vi "Format CSV.vi"(8 "error in (no error)":errorcluster, 9 "delimiter":string=",", 10 "CSV File Input":path, 11 "Original CSV Format":enum16{"Format A", "Format B"}(ring)) -> (0 "error out":errorcluster, 1 "Parcel Length":i32[](array[numeric]), 2 "All Terminal Data":T1(array[cluster]))   [LabVIEW 2017] (continued)
"30:40.9", "30:41.0", "30:41.0", "30:41.0", "30:41.1", "30:41.1", "30:41.1", "30:41.2", "30:41.2", "30:41.2", "30:41.3", "30:41.3", "30:41.3", "30:41.4", "30:41.4", "30:41.4", "30:41.5", "30:41.5", "30:41.5", "30:41.6", "30:41.6", "30:41.6", "30:41.7", "30:41.7", "30:41.7", "30:41.8", "30:41.8", "30:41.8", "30:41.9", "30:41.9", "30:41.9", "30:42.0", "30:42.0", "30:42.0", "30:42.1", "30:42.1", "30:42.1", "30:42.2", "30:42.2", "30:42.2", "30:42.3", "30:42.3", "30:42.3", "30:42.4", "30:42.4", "30:42.4", "30:42.5", "30:42.5", "30:42.5", "30:42.6", "30:42.6", "30:42.6", "30:42.7", "30:42.7", "30:42.7", "30:42.8", "30:42.8", "30:42.8", "30:42.9", "30:42.9", "30:42.9", "30:43.0", "30:43.0", "30:43.0", "30:43.1", "30:43.1", "30:43.1", "30:43.2", "30:43.2", "30:43.2", "30:43.3", "30:43.3", "30:43.3", "30:43.4", "30:43.4", "30:43.4", "30:43.5", "30:43.5", "30:43.5", "30:43.6", "30:43.6", "30:43.6", "30:43.7", "30:43.7", "30:43.7", "30:43.8", "30:43.8", "30:43.8", "30:43.9", "30:43.9", "30:43.9", "30:44.0", "30:44.0", "30:44.0", "30:44.1", "30:44.1", "30:44.1", "30:44.2", "30:44.2", "30:44.2", "30:44.3", "30:44.3", "30:44.3", "30:44.4", "30:44.4", "30:44.4", "30:44.5", "30:44.5", "30:44.5", "30:44.6", "30:44.6", "30:44.6", "30:44.7", "30:44.7", "30:44.7", "30:44.8", "30:44.8", "30:44.8", "30:44.9", "30:44.9", "30:44.9", "30:45.0", "30:45.0", "30:45.0", "30:45.1", "30:45.1", "30:45.1", "30:45.2", "30:45.2", "30:45.2", "30:45.3", "30:45.3", "30:45.3", "30:45.4", "30:45.4", "30:45.4", "30:45.5", "30:45.5", "30:45.5", "30:45.6", "30:45.6", "30:45.6", "30:45.7", "30:45.7", "30:45.7", "30:45.8", "30:45.8", "30:45.8", "30:45.9", "30:45.9", "30:45.9", "30:46.0", "30:46.0", "30:46.0", "30:46.1", "30:46.1", "30:46.1", "30:46.2", "30:46.2", "30:46.2", "30:46.3", "30:46.3", "30:46.3", "30:46.4", "30:46.4", "30:46.4", "30:46.5", "30:46.5", "30:46.5", "30:46.6", "30:46.6", "30:46.6", "30:46.7", "30:46.7", "30:46.7", "30:46.8", "30:46.8", "30:46.8", "30:46.9", "30:46.9", "30:46.9", "30:47.0", "30:47.0", "30:47.0", "30:47.1", "30:47.1", "30:47.1", "30:47.2", "30:47.2", "30:47.2", "30:47.3", "30:47.3", "30:47.3", "30:47.4", "30:47.4", "30:47.4", "30:47.5", "30:47.5", "30:47.5", "30:47.6", "30:47.6", "30:47.6", "30:47.7", "30:47.7", "30:47.7", "30:47.8", "30:47.8", "30:47.8", "30:47.9", "30:47.9", "30:47.9", "30:48.0", "30:48.0", "30:48.0", "30:48.1", "30:48.1", "30:48.1", "30:48.2", "30:48.2", "30:48.2", "30:48.3", "30:48.3", "30:48.3", "30:48.4", "30:48.4", "30:48.4", "30:48.5", "30:48.5", "30:48.5", "30:48.6", "30:48.6", "30:48.6", "30:48.7", "30:48.7", "30:48.7", "30:48.8", "30:48.8", "30:48.8", "30:48.9", "30:48.9", "30:48.9", "30:49.0", "30:49.0", "30:49.0", "30:49.1", "30:49.1", "30:49.1", "30:49.2", "30:49.2", "30:49.2", "30:49.3", "30:49.3", "30:49.3", "30:49.4", "30:49.4", "30:49.4", "30:49.5", "30:49.5", "30:49.5", "30:49.6", "30:49.6", "30:49.6", "30:49.7", "30:49.7", "30:49.7", "30:49.8", "30:49.8", "30:49.8", "30:49.9", "30:49.9", "30:49.9", "30:50.0", "30:50.0", "30:50.0", "30:50.1", "30:50.1", "30:50.1", "30:50.2", "30:50.2", "30:50.2", "30:50.3", "30:50.3", "30:50.3", "30:50.4", "30:50.4", "30:50.4", "30:50.5", "30:50.5", "30:50.5", "30:50.6", "30:50.6", "30:50.6", "30:50.7", "30:50.7", "30:50.7", "30:50.8", "30:50.8", "30:50.8", "30:50.9", "30:50.9", "30:50.9", "30:51.0", "30:51.0", "30:51.0", "30:51.1", "30:51.1", "30:51.1", "30:51.2", "30:51.2", "30:51.2", "30:51.3", "30:51.3", "30:51.3", "30:51.4", "30:51.4", "30:51.4", "30:51.5", "30:51.5", "30:51.5", "30:51.6", "30:51.6", "30:51.6", "30:51.7", "30:51.7", "30:51.7", "30:51.8", "30:51.8", "30:51.8", "30:51.9", "30:51.9", "30:51.9", "30:52.0", "30:52.0", "30:52.0", "30:52.1", "30:52.1", "30:52.1", "30:52.2", "30:52.2", "30:52.2", "30:52.3", "30:52.3", "30:52.3", "30:52.4", "30:52.4", "30:52.4", "30:52.5", "30:52.5", "30:52.5", "30:52.6", "30:52.6", "30:52.6", "30:52.7", "30:52.7", "30:52.7", "30:52.8", "30:52.8", "30:52.8", "30:52.9", "30:52.9", "30:52.9", "30:53.0", "30:53.0", "30:53.0", "30:53.1", "30:53.1", "30:53.1", "30:53.2", "30:53.2", "30:53.2", "30:53.3", "30:53.3", "30:53.3", "30:53.4", "30:53.4", "30:53.4", "30:53.5", "30:53.5", "30:53.5", "30:53.6", "30:53.6", "30:53.6", "30:53.7", "30:53.7", "30:53.7", "30:53.8", "30:53.8", "30:53.8", "30:53.9", "30:53.9", "30:53.9", "30:54.0", "30:54.0", "30:54.0", "30:54.1", "30:54.1", "30:54.1", "30:54.2", "30:54.2", "30:54.2", "30:54.3", "30:54.3", "30:54.3", "30:54.4", "30:54.4", "30:54.4", "30:54.5", "30:54.5", "30:54.5", "30:54.6", "30:54.6", "30:54.6", "30:54.7", "30:54.7", "30:54.7", "30:54.8", "30:54.8", "30:54.8", "30:54.9", "30:54.9", "30:54.9", "30:55.0", "30:55.0", "30:55.0", "30:55.1", "30:55.1", "30:55.1", "30:55.2", "30:55.2", "30:55.2", "30:55.3", "30:55.3", "30:55.3", "30:55.4", "30:55.4", "30:55.4", "30:55.5", "30:55.5", "30:55.5", "30:55.6", "30:55.6", "30:55.6", "30:55.7", "30:55.7", "30:55.7", "30:55.8", "30:55.8", "30:55.8", "30:55.9", "30:55.9", "30:55.9", "30:56.0", "30:56.0", "30:56.0", "30:56.1", "30:56.1", "30:56.1", "30:56.2", "30:56.2", "30:56.2", "30:56.3", "30:56.3", "30:56.3", "30:56.4", "30:56.4", "30:56.4", "30:56.5", "30:56.5", "30:56.5", "30:56.6", "30:56.6", "30:56.6", "30:56.7", "30:56.7", "30:56.7", "30:56.8", "30:56.8", "30:56.8", "30:56.9", "30:56.9", "30:56.9", "30:57.0", "30:57.0", "30:57.0", "30:57.1", "30:57.1", "30:57.1", "30:57.2", "30:57.2", "30:57.2", "30:57.3", "30:57.3", "30:57.3", "30:57.4", "30:57.4", "30:57.4", "30:57.5", "30:57.5", "30:57.5", "30:57.6", "30:57.6", "30:57.6", "30:57.7", "30:57.7", "30:57.7", "30:57.8", "30:57.8", "30:57.8", "30:57.9", "30:57.9", "30:57.9", "30:58.0", "30:58.0", "30:58.0", "30:58.1", "30:58.1", "30:58.1", "30:58.2", "30:58.2", "30:58.2", "30:58.3", "30:58.3", "30:58.3", "30:58.4", "30:58.4", "30:58.4", "30:58.5", "30:58.5", "30:58.5", "30:58.6", "30:58.6", "30:58.6", "30:58.7", "30:58.7", "30:58.7", "30:58.8", "30:58.8", "30:58.8", "30:58.9", "30:58.9", "30:58.9", "30:59.0", "30:59.0", "30:59.0", "30:59.1", "30:59.1", "30:59.1", "30:59.2", "30:59.2", "30:59.2", "30:59.3", "30:59.3", "30:59.3", "30:59.4", "30:59.4", "30:59.4", "30:59.5", "30:59.5", "30:59.5", "30:59.6", "30:59.6", "30:59.6", "30:59.7", "30:59.7", "30:59.7", "30:59.8", "30:59.8", "30:59.8", "30:59.9", "30:59.9", "30:59.9", "31:00.0", "31:00.0", "31:00.0", "31:00.1", "31:00.1", "31:00.1", "31:00.2", "31:00.2", "31:00.2", "31:00.3", "31:00.3", "31:00.3", "31:00.4", "31:00.4", "31:00.4", "31:00.5", "31:00.5", "31:00.5", "31:00.6", "31:00.6", "31:00.6", "31:00.7", "31:00.7", "31:00.7", "31:00.8", "31:00.8", "31:00.8", "31:00.9", "31:00.9", "31:00.9", "31:01.0", "31:01.0", "31:01.0", "31:01.1", "31:01.1", "31:01.1", "31:01.2", "31:01.2", "31:01.2", "31:01.3", "31:01.3", "31:01.3", "31:01.4", "31:01.4", "31:01.4", "31:01.5", "31:01.5", "31:01.5", "31:01.6", "31:01.6", "31:01.6", "31:01.7", "31:01.7", "31:01.7", "31:01.8", "31:01.8", "31:01.8", "31:01.9", "31:01.9", "31:01.9", "31:02.0", "31:02.0", "31:02.0", "31:02.1", "31:02.1", "31:02.1", "31:02.2", "31:02.2", "31:02.2", "31:02.3", "31:02.3", "31:02.3", "31:02.4", "31:02.4", "31:02.4", "31:02.5", "31:02.5", "31:02.5", "31:02.6", "31:02.6", "31:02.6", "31:02.7", "31:02.7", "31:02.7", "31:02.8", "31:02.8", "31:02.8", "31:02.9", "31:02.9", "31:02.9", "31:03.0", "31:03.0", "31:03.0", "31:03.1", "31:03.1", "31:03.1", "31:03.2", "31:03.2", "31:03.2", "31:03.3", "31:03.3", "31:03.3", "31:03.4", "31:03.4", "31:03.4", "31:03.5", "31:03.5", "31:03.5", "31:03.6", "31:03.6", "31:03.6", "31:03.7", "31:03.7", "31:03.7", "31:03.8", "31:03.8", "31:03.8", "31:03.9", "31:03.9", "31:03.9", "31:04.0", "31:04.0", "31:04.0", "31:04.1", "31:04.1", "31:04.1", "31:04.2", "31:04.2", "31:04.2", "31:04.3", "31:04.3", "31:04.3", "31:04.4", "31:04.4", "31:04.4", "31:04.5", "31:04.5", "31:04.5", "31:04.6", "31:04.6", "31:04.6", "31:04.7", "31:04.7", "31:04.7", "31:04.8", "31:04.8", "31:04.8", "31:04.9", "31:04.9", "31:04.9", "31:05.0", "31:05.0", "31:05.0", "31:05.1", "31:05.1", "31:05.1", "31:05.2", "31:05.2", "31:05.2", "31:05.3", "31:05.3", "31:05.3", "31:05.4", "31:05.4", "31:05.4", "31:05.5", "31:05.5", "31:05.5", "31:05.6", "31:05.6", "31:05.6", "31:05.7", "31:05.7", "31:05.7", "31:05.8", "31:05.8", "31:05.8", "31:05.9", "31:05.9", "31:05.9", "31:06.0", "31:06.0", "31:06.0", "31:06.1", "31:06.1", "31:06.1", "31:06.2", "31:06.2", "31:06.2", "31:06.3", "31:06.3", "31:06.3", "31:06.4", "31:06.4", "31:06.4", "31:06.5", "31:06.5", "31:06.5", "31:06.6", "31:06.6", "31:06.6", "31:06.7", "31:06.7", "31:06.7", "31:06.8", "31:06.8", "31:06.8", "31:06.9", "31:06.9", "31:06.9", "31:07.0", "31:07.0", "31:07.0", "31:07.1", "31:07.1", "31:07.1", "31:07.2", "31:07.2", "31:07.2", "31:07.3", "31:07.3", "31:07.3", "31:07.4", "31:07.4", "31:07.4", "31:07.5", "31:07.5", "31:07.5", "31:07.6", "31:07.6", "31:07.6", "31:07.7", "31:07.7", "31:07.7", "31:07.8", "31:07.8", "31:07.8", "31:07.9", "31:07.9", "31:07.9", "31:08.0", "31:08.0", "31:08.0", "31:08.1", "31:08.1", "31:08.1", "31:08.2", "31:08.2", "31:08.2", "31:08.3", "31:08.3", "31:08.3", "31:08.4", "31:08.4", "31:08.4", "31:08.5", "31:08.5", "31:08.5", "31:08.6", "31:08.6", "31:08.6", "31:08.7", "31:08.7", "31:08.7", "31:08.8", "31:08.8", "31:08.8", "31:08.9", "31:08.9", "31:08.9", "31:09.0", "31:09.0", "31:09.0", "31:09.1", "31:09.1", "31:09.1", "31:09.2", "31:09.2", "31:09.2", "31:09.3", "31:09.3", "31:09.3", "31:09.4", "31:09.4", "31:09.4", "31:09.5", "31:09.5", "31:09.5", "31:09.6", "31:09.6", "31:09.6", "31:09.7", "31:09.7", "31:09.7", "31:09.8", "31:09.8", "31:09.8", "31:09.9", "31:09.9", "31:09.9", "31:10.0", "31:10.0", "31:10.0", "31:10.1", "31:10.1", "31:10.1", "31:10.2", "31:10.2", "31:10.2", "31:10.3", "31:10.3", "31:10.3", "31:10.4", "31:10.4", "31:10.4", "31:10.5", "31:10.5", "31:10.5", "31:10.6", "31:10.6", "31:10.6", "31:10.7", "31:10.7", "31:10.7", "31:10.8", "31:10.8", "31:10.8", "31:10.9", "31:10.9", "31:10.9", "31:11.0", "31:11.0", "31:11.0", "31:11.1", "31:11.1", "31:11.1", "31:11.2", "31:11.2", "31:11.2", "31:11.3", "31:11.3", "31:11.3", "31:11.4", "31:11.4", "31:11.4", "31:11.5", "31:11.5", "31:11.5", "31:11.6", "31:11.6", "31:11.6", "31:11.7", "31:11.7", "31:11.7", "31:11.8", "31:11.8", "31:11.8", "31:11.9", "31:11.9", "31:11.9", "31:12.0", "31:12.0", "31:12.0", "31:12.1", "31:12.1", "31:12.1", "31:12.2", "31:12.2", "31:12.2", "31:12.3", "31:12.3", "31:12.3", "31:12.4", "31:12.4", "31:12.4", "31:12.5", "31:12.5", "31:12.5", "31:12.6", "31:12.6", "31:12.6", "31:12.7", "31:12.7", "31:12.7", "31:12.8", "31:12.8", "31:12.8", "31:12.9", "31:12.9", "31:12.9", "31:13.0", "31:13.0", "31:13.0", "31:13.1", "31:13.1", "31:13.1", "31:13.2", "31:13.2", "31:13.2", "31:13.3", "31:13.3", "31:13.3", "31:13.4", "31:13.4", "31:13.4", "31:13.5", "31:13.5", "31:13.5", "31:13.6", "31:13.6", "31:13.6", "31:13.7", "31:13.7", "31:13.7", "31:13.8", "31:13.8", "31:13.8", "31:13.9", "31:13.9", "31:13.9", "31:14.0", "31:14.0", "31:14.0", "31:14.1", "31:14.1", "31:14.1", "31:14.2", "31:14.2", "31:14.2", "31:14.3", "31:14.3", "31:14.3", "31:14.4", "31:14.4", "31:14.4", "31:14.5", "31:14.5", "31:14.5", "31:14.6", "31:14.6", "31:14.6", "31:14.7", "31:14.7", "31:14.7", "31:14.8", "31:14.8", "31:14.8", "31:14.9", "31:14.9", "31:14.9", "31:15.0", "31:15.0", "31:15.0", "31:15.1", "31:15.1", "31:15.1", "31:15.2", "31:15.2", "31:15.2", "31:15.3", "31:15.3", "31:15.3", "31:15.4", "31:15.4", "31:15.4", "31:15.5", "31:15.5", "31:15.5", "31:15.6", "31:15.6", "31:15.6", "31:15.7", "31:15.7", "31:15.7", "31:15.8", "31:15.8", "31:15.8", "31:15.9", "31:15.9", "31:15.9", "31:16.0", "31:16.0", "31:16.0", "31:16.1", "31:16.1", "31:16.1", "31:16.2", "31:16.2", "31:16.2", "31:16.3", "31:16.3", "31:16.3", "31:16.4", "31:16.4", "31:16.4", "31:16.5", "31:16.5", "31:16.5", "31:16.6", "31:16.6", "31:16.6", "31:16.7", "31:16.7", "31:16.7", "31:16.8", "31:16.8", "31:16.8", "31:16.9", "31:16.9", "31:16.9", "31:17.0", "31:17.0", "31:17.0", "31:17.1", "31:17.1", "31:17.1", "31:17.2", "31:17.2", "31:17.2", "31:17.3", "31:17.3", "31:17.3", "31:17.4", "31:17.4", "31:17.4", "31:17.5", "31:17.5", "31:17.5", "31:17.6", "31:17.6", "31:17.6", "31:17.7", "31:17.7", "31:17.7", "31:17.8", "31:17.8", "31:17.8", "31:17.9", "31:17.9", "31:17.9", "31:18.0", "31:18.0", "31:18.0", "31:18.1", "31:18.1", "31:18.1", "31:18.2", "31:18.2", "31:18.2", "31:18.3", "31:18.3", "31:18.3", "31:18.4", "31:18.4", "31:18.4", "31:18.5", "31:18.5", "31:18.5", "31:18.6", "31:18.6", "31:18.6", "31:18.7", "31:18.7", "31:18.7", "31:18.8", "31:18.8", "31:18.8", "31:18.9", "31:18.9", "31:18.9", "31:19.0", "31:19.0", "31:19.0", "31:19.1", "31:19.1", "31:19.1", "31:19.2", "31:19.2", "31:19.2", "31:19.3", "31:19.3", "31:19.3", "31:19.4", "31:19.4", "31:19.4", "31:19.5", "31:19.5", "31:19.5", "31:19.6", "31:19.6", "31:19.6", "31:19.7", "31:19.7", "31:19.7", "31:19.8", "31:19.8", "31:19.8", "31:19.9", "31:19.9", "31:19.9", "31:20.0", "31:20.0", "31:20.0", "31:20.1", "31:20.1", "31:20.1", "31:20.2", "31:20.2", "31:20.2", "31:20.3", "31:20.3", "31:20.3", "31:20.4", "31:20.4", "31:20.4", "31:20.5", "31:20.5", "31:20.5", "31:20.6", "31:20.6", "31:20.6", "31:20.7", "31:20.7", "31:20.7", "31:20.8", "31:20.8", "31:20.8", "31:20.9", "31:20.9", "31:20.9", "31:21.0", "31:21.0", "31:21.0", "31:21.1", "31:21.1", "31:21.1", "31:21.2", "31:21.2", "31:21.2", "31:21.3", "31:21.3", "31:21.3", "31:21.4", "31:21.4", "31:21.4", "31:21.5", "31:21.5", "31:21.5", "31:21.6", "31:21.6", "31:21.6", "31:21.7", "31:21.7", "31:21.7", "31:21.8", "31:21.8", "31:21.8", "31:21.9", "31:21.9", "31:21.9", "31:22.0", "31:22.0", "31:22.0", "31:22.1", "31:22.1", "31:22.1", "31:22.2", "31:22.2", "31:22.2", "31:22.3", "31:22.3", "31:22.3", "31:22.4", "31:22.4", "31:22.4", "31:22.5", "31:22.5", "31:22.5", "31:22.6", "31:22.6", "31:22.6", "31:22.7", "31:22.7", "31:22.7", "31:22.8", "31:22.8", "31:22.8", "31:22.9", "31:22.9", "31:22.9", "31:23.0", "31:23.0", "31:23.0", "31:23.1", "31:23.1", "31:23.1", "31:23.2", "31:23.2", "31:23.2", "31:23.3", "31:23.3", "31:23.3", "31:23.4", "31:23.4", "31:23.4", "31:23.5", "31:23.5", "31:23.5", "31:23.6", "31:23.6", "31:23.6", "31:23.7", "31:23.7", "31:23.7", "31:23.8", "31:23.8", "31:23.8", "31:23.9", "31:23.9", "31:23.9", "31:24.0", "31:24.0", "31:24.0", "31:24.1", "31:24.1", "31:24.1", "31:24.2", "31:24.2", "31:24.2", "31:24.3", "31:24.3", "31:24.3", "31:24.4", "31:24.4", "31:24.4", "31:24.5", "31:24.5", "31:24.5", "31:24.6", "31:24.6", "31:24.6", "31:24.7", "31:24.7", "31:24.7", "31:24.8", "31:24.8", "31:24.8", "31:24.9", "31:24.9", "31:24.9", "31:25.0", "31:25.0", "31:25.0", "31:25.1", "31:25.1", "31:25.1", "31:25.2", "31:25.2", "31:25.2", "31:25.3", "31:25.3", "31:25.3", "31:25.4", "31:25.4", "31:25.4", "31:25.5", "31:25.5", "31:25.5", "31:25.6", "31:25.6", "31:25.6", "31:25.7", "31:25.7", "31:25.7", "31:25.8", "31:25.8", "31:25.8", "31:25.9", "31:25.9", "31:25.9", "31:26.0", "31:26.0", "31:26.0", "31:26.1", "31:26.1", "31:26.1", "31:26.2", "31:26.2", "31:26.2", "31:26.3", "31:26.3", "31:26.3", "31:26.4", "31:26.4", "31:26.4", "31:26.5", "31:26.5", "31:26.5", "31:26.6", "31:26.6", "31:26.6", "31:26.7", "31:26.7", "31:26.7", "31:26.8", "31:26.8", "31:26.8", "31:26.9", "31:26.9", "31:26.9", "31:27.0", "31:27.0", "31:27.0", "31:27.1", "31:27.1", "31:27.1", "31:27.2", "31:27.2", "31:27.2", "31:27.3", "31:27.3", "31:27.3", "31:27.4", "31:27.4", "31:27.4", "31:27.5", "31:27.5", "31:27.5", "31:27.6", "31:27.6", "31:27.6", "31:27.7", "31:27.7", "31:27.7", "31:27.8", "31:27.8", "31:27.8", "31:27.9", "31:27.9", "31:27.9", "31:28.0", "31:28.0", "31:28.0", "31:28.1", "31:28.1", "31:28.1", "31:28.2", "31:28.2", "31:28.2", "31:28.3", "31:28.3", "31:28.3", "31:28.4", "31:28.4", "31:28.4", "31:28.5", "31:28.5", "31:28.5", "31:28.6", "31:28.6", "31:28.6", "31:28.7", "31:28.7", "31:28.7", "31:28.8", "31:28.8", "31:28.8", "31:28.9", "31:28.9", "31:28.9", "31:29.0", "31:29.0", "31:29.0", "31:29.1", "31:29.1", "31:29.1", "31:29.2", "31:29.2", "31:29.2", "31:29.3", "31:29.3", "31:29.3", "31:29.4", "31:29.4", "31:29.4", "31:29.5", "31:29.5", "31:29.5", "31:29.6", "31:29.6", "31:29.6", "31:29.7", "31:29.7", "31:29.7", "31:29.8", "31:29.8", "31:29.8", "31:29.9", "31:29.9", "31:29.9", "31:30.0", "31:30.0", "31:30.0", "31:30.1", "31:30.1", "31:30.1", "31:30.2", "31:30.2", "31:30.2", "31:30.3", "31:30.3", "31:30.3", "31:30.4", "31:30.4", "31:30.4", "31:30.5", "31:30.5", "31:30.5", "31:30.6", "31:30.6", "31:30.6", "31:30.7", "31:30.7", "31:30.7", "31:30.8", "31:30.8", "31:30.8", "31:30.9", "31:30.9", "31:30.9", "31:31.0", "31:31.0", "31:31.0", "31:31.1", "31:31.1", "31:31.1", "31:31.2", "31:31.2", "31:31.2", "31:31.3", "31:31.3", "31:31.3", "31:31.4", "31:31.4", "31:31.4", "31:31.5", "31:31.5", "31:31.5", "31:31.6", "31:31.6", "31:31.6", "31:31.7", "31:31.7", "31:31.7", "31:31.8", "31:31.8", "31:31.8", "31:31.9", "31:31.9", "31:31.9", "31:32.0", "31:32.0", "31:32.0", "31:32.1", "31:32.1", "31:32.1", "31:32.2", "31:32.2", "31:32.2", "31:32.3", "31:32.3", "31:32.3", "31:32.4", "31:32.4", "31:32.4", "31:32.5", "31:32.5", "31:32.5", "31:32.6", "31:32.6", "31:32.6", "31:32.7", "31:32.7", "31:32.7", "31:32.8", "31:32.8", "31:32.8", "31:32.9", "31:32.9", "31:32.9", "31:33.0", "31:33.0", "31:33.0", "31:33.1", "31:33.1", "31:33.1", "31:33.2", "31:33.2", "31:33.2", "31:33.3", "31:33.3", "31:33.3", "31:33.4", "31:33.4", "31:33.4", "31:33.5", "31:33.5", "31:33.5", "31:33.6", "31:33.6", "31:33.6", "31:33.7", "31:33.7", "31:33.7", "31:33.8", "31:33.8", "31:33.8", "31:33.9", "31:33.9", "31:33.9", "31:34.0", "31:34.0", "31:34.0", "31:34.1", "31:34.1", "31:34.1", "31:34.2", "31:34.2", "31:34.2", "31:34.3", "31:34.3", "31:34.3", "31:34.4", "31:34.4", "31:34.4", "31:34.5", "31:34.5", "31:34.5", "31:34.6", "31:34.6", "31:34.6", "31:34.7", "31:34.7", "31:34.7", "31:34.8", "31:34.8", "31:34.8", "31:34.9", "31:34.9", "31:34.9", "31:35.0", "31:35.0", "31:35.0", "31:35.1", "31:35.1", "31:35.1", "31:35.2", "31:35.2", "31:35.2", "31:35.3", "31:35.3", "31:35.3", "31:35.4", "31:35.4", "31:35.4", "31:35.5", "31:35.5", "31:35.5", "31:35.6", "31:35.6", "31:35.6", "31:35.7", "31:35.7", "31:35.7", "31:35.8", "31:35.8", "31:35.8", "31:35.9", "31:35.9", "31:35.9", "31:36.0", "31:36.0", "31:36.0", "31:36.1", "31:36.1", "31:36.1", "31:36.2", "31:36.2", "31:36.2", "31:36.3", "31:36.3", "31:36.3", "31:36.4", "31:36.4", "31:36.4", "31:36.5", "31:36.5", "31:36.5", "31:36.6", "31:36.6", "31:36.6", "31:36.7", "31:36.7", "31:36.7", "31:36.8", "31:36.8", "31:36.8", "31:36.9", "31:36.9", "31:36.9", "31:37.0", "31:37.0", "31:37.0", "31:37.1", "31:37.1", "31:37.1", "31:37.2", "31:37.2", "31:37.2", "31:37.3", "31:37.3", "31:37.3", "31:37.4", "31:37.4", "31:37.4", "31:37.5", "31:37.5", "31:37.5", "31:37.6", "31:37.6", "31:37.6", "31:37.7", "31:37.7", "31:37.7", "31:37.8", "31:37.8", "31:37.8", "31:37.9", "31:37.9", "31:37.9", "31:38.0", "31:38.0", "31:38.0", "31:38.1", "31:38.1", "31:38.1", "31:38.2", "31:38.2", "31:38.2", "31:38.3", "31:38.3", "31:38.3", "31:38.4", "31:38.4", "31:38.4", "31:38.5", "31:38.5", "31:38.5", "31:38.6", "31:38.6", "31:38.6", "31:38.7", "31:38.7", "31:38.7", "31:38.8", "31:38.8", "31:38.8", "31:38.9", "31:38.9", "31:38.9", "31:39.0", "31:39.0", "31:39.0", "31:39.1", "31:39.1", "31:39.1", "31:39.2", "31:39.2", "31:39.2", "31:39.3", "31:39.3", "31:39.3", "31:39.4", "31:39.4", "31:39.4", "31:39.5", "31:39.5", "31:39.5", "31:39.6", "31:39.6", "31:39.6", "31:39.7", "31:39.7", "31:39.7", "31:39.8", "31:39.8", "31:39.8", "31:39.9", "31:39.9", "31:39.9", "31:40.0", "31:40.0", "31:40.0", "31:40.1", "31:40.1", "31:40.1", "31:40.2", "31:40.2", "31:40.2", "31:40.3", "31:40.3", "31:40.3", "31:40.4", "31:40.4", "31:40.4", "31:40.5", "31:40.5", "31:40.5", "31:40.6", "31:40.6", "31:40.6", "31:40.7", "31:40.7", "31:40.7", "31:40.8", "31:40.8", "31:40.8", "31:40.9", "31:40.9", "31:40.9", "31:41.0", "31:41.0", "31:41.0", "31:41.1", "31:41.1", "31:41.1", "31:41.2", "31:41.2", "31:41.2", "31:41.3", "31:41.3", "31:41.3", "31:41.4", "31:41.4", "31:41.4", "31:41.5", "31:41.5", "31:41.5", "31:41.6", "31:41.6", "31:41.6", "31:41.7", "31:41.7", "31:41.7", "31:41.8", "31:41.8", "31:41.8", "31:41.9", "31:41.9", "31:41.9", "31:42.0", "31:42.0", "31:42.0", "31:42.1", "31:42.1", "31:42.1", "31:42.2", "31:42.2", "31:42.2", "31:42.3", "31:42.3", "31:42.3", "31:42.4", "31:42.4", "31:42.4", "31:42.5", "31:42.5", "31:42.5", "31:42.6", "31:42.6", "31:42.6", "31:42.7", "31:42.7", "31:42.7", "31:42.8", "31:42.8", "31:42.8", "31:42.9", "31:42.9", "31:42.9", "31:43.0", "31:43.0", "31:43.0", "31:43.1", "31:43.1", "31:43.1", "31:43.2", "31:43.2", "31:43.2", "31:43.3", "31:43.3", "31:43.3", "31:43.4", "31:43.4", "31:43.4", "31:43.5", "31:43.5", "31:43.5", "31:43.6", "31:43.6", "31:43.6", "31:43.7", "31:43.7", "31:43.7", "31:43.8", "31:43.8", "31:43.8", "31:43.9", "31:43.9", "31:43.9", "31:44.0", "31:44.0", "31:44.0", "31:44.1", "31:44.1", "31:44.1", "31:44.2", "31:44.2", "31:44.2", "31:44.3", "31:44.3", "31:44.3", "31:44.4", "31:44.4", "31:44.4", "31:44.5", "31:44.5", "31:44.5", "31:44.6", "31:44.6", "31:44.6", "31:44.7", "31:44.7", "31:44.7", "31:44.8", "31:44.8", "31:44.8", "31:44.9", "31:44.9", "31:44.9", "31:45.0", "31:45.0", "31:45.0", "31:45.1", "31:45.1", "31:45.1", "31:45.2", "31:45.2", "31:45.2", "31:45.3", "31:45.3", "31:45.3", "31:45.4", "31:45.4", "31:45.4", "31:45.5", "31:45.5", "31:45.5", "31:45.6", "31:45.6", "31:45.6", "31:45.7", "31:45.7", "31:45.7", "31:45.8", "31:45.8", "31:45.8", "31:45.9", "31:45.9", "31:45.9", "31:46.0", "31:46.0", "31:46.0", "31:46.1", "31:46.1", "31:46.1", "31:46.2", "31:46.2", "31:46.2", "31:46.3", "31:46.3", "31:46.3", "31:46.4", "31:46.4", "31:46.4", "31:46.5", "31:46.5", "31:46.5", "31:46.6", "31:46.6", "31:46.6", "31:46.7", "31:46.7", "31:46.7", "31:46.8", "31:46.8", "31:46.8", "31:46.9", "31:46.9", "31:46.9", "31:47.0", "31:47.0", "31:47.0", "31:47.1", "31:47.1", "31:47.1", "31:47.2", "31:47.2", "31:47.2", "31:47.3", "31:47.3", "31:47.3", "31:47.4", "31:47.4", "31:47.4", "31:47.5", "31:47.5", "31:47.5", "31:47.6", "31:47.6", "31:47.6", "31:47.7", "31:47.7", "31:47.7", "31:47.8", "31:47.8", "31:47.8", "31:47.9", "31:47.9", "31:47.9", "31:48.0", "31:48.0", "31:48.0", "31:48.1", "31:48.1", "31:48.1", "31:48.2", "31:48.2", "31:48.2", "31:48.3", "31:48.3", "31:48.3", "31:48.4", "31:48.4", "31:48.4", "31:48.5", "31:48.5", "31:48.5", "31:48.6", "31:48.6", "31:48.6", "31:48.7", "31:48.7", "31:48.7", "31:48.8", "31:48.8", "31:48.8", "31:48.9", "31:48.9", "31:48.9", "31:49.0", "31:49.0", "31:49.0", "31:49.1", "31:49.1", "31:49.1", "31:49.2", "31:49.2", "31:49.2", "31:49.3", "31:49.3", "31:49.3", "31:49.4", "31:49.4", "31:49.4", "31:49.5", "31:49.5", "31:49.5", "31:49.6", "31:49.6", "31:49.6", "31:49.7", "31:49.7", "31:49.7", "31:49.8", "31:49.8", "31:49.8", "31:49.9", "31:49.9", "31:49.9", "31:50.0", "31:50.0", "31:50.0", "31:50.1", "31:50.1", "31:50.1", "31:50.2", "31:50.2", "31:50.2", "31:50.3", "31:50.3", "31:50.3", "31:50.4", "31:50.4", "31:50.4", "31:50.5", "31:50.5", "31:50.5", "31:50.6", "31:50.6", "31:50.6", "31:50.7", "31:50.7", "31:50.7", "31:50.8", "31:50.8", "31:50.8", "31:50.9", "31:50.9", "31:50.9", "31:51.0", "31:51.0", "31:51.0", "31:51.1", "31:51.1", "31:51.1", "31:51.2", "31:51.2", "31:51.2", "31:51.3", "31:51.3", "31:51.3", "31:51.4", "31:51.4", "31:51.4", "31:51.5", "31:51.5", "31:51.5", "31:51.6", "31:51.6", "31:51.6", "31:51.7", "31:51.7", "31:51.7", "31:51.8", "31:51.8", "31:51.8", "31:51.9", "31:51.9", "31:51.9", "31:52.0", "31:52.0", "31:52.0", "31:52.1", "31:52.1", "31:52.1", "31:52.2", "31:52.2", "31:52.2", "31:52.3", "31:52.3", "31:52.3", "31:52.4", "31:52.4", "31:52.4", "31:52.5", "31:52.5", "31:52.5", "31:52.6", "31:52.6", "31:52.6", "31:52.7", "31:52.7", "31:52.7", "31:52.8", "31:52.8", "31:52.8", "31:52.9", "31:52.9", "31:52.9", "31:53.0", "31:53.0", "31:53.0", "31:53.1", "31:53.1", "31:53.1", "31:53.2", "31:53.2", "31:53.2", "31:53.3", "31:53.3", "31:53.3", "31:53.4", "31:53.4", "31:53.4", "31:53.5", "31:53.5", "31:53.5", "31:53.6", "31:53.6", "31:53.6", "31:53.7", "31:53.7", "31:53.7", "31:53.8", "31:53.8", "31:53.8", "31:53.9", "31:53.9", "31:53.9", "31:54.0", "31:54.0", "31:54.0", "31:54.1", "31:54.1", "31:54.1", "31:54.2", "31:54.2", "31:54.2", "31:54.3", "31:54.3", "31:54.3", "31:54.4", "31:54.4", "31:54.4", "31:54.5", "31:54.5", "31:54.5", "31:54.6", "31:54.6", "31:54.6", "31:54.7", "31:54.7", "31:54.7", "31:54.8", "31:54.8", "31:54.8", "31:54.9", "31:54.9", "31:54.9", "31:55.0", "31:55.0", "31:55.0", "31:55.1", "31:55.1", "31:55.1", "31:55.2", "31:55.2", "31:55.2", "31:55.3", "31:55.3", "31:55.3", "31:55.4", "31:55.4", "31:55.4", "31:55.5", "31:55.5", "31:55.5", "31:55.6", "31:55.6", "31:55.6", "31:55.7", "31:55.7", "31:55.7", "31:55.8", "31:55.8", "31:55.8", "31:55.9", "31:55.9", "31:55.9", "31:56.0", "31:56.0", "31:56.0", "31:56.1", "31:56.1", "31:56.1", "31:56.2", "31:56.2", "31:56.2", "31:56.3", "31:56.3", "31:56.3", "31:56.4", "31:56.4", "31:56.4", "31:56.5", "31:56.5", "31:56.5", "31:56.6", "31:56.6", "31:56.6", "31:56.7", "31:56.7", "31:56.7", "31:56.8", "31:56.8", "31:56.8", "31:56.9", "31:56.9", "31:56.9", "31:57.0", "31:57.0", "31:57.0", "31:57.1", "31:57.1", "31:57.1", "31:57.2", "31:57.2", "31:57.2", "31:57.3", "31:57.3", "31:57.3", "31:57.4", "31:57.4", "31:57.4", "31:57.5", "31:57.5", "31:57.5", "31:57.6", "31:57.6", "31:57.6", "31:57.7", "31:57.7", "31:57.7", "31:57.8", "31:57.8", "31:57.8", "31:57.9", "31:57.9", "31:57.9", "31:58.0", "31:58.0", "31:58.0", "31:58.1", "31:58.1", "31:58.1", "31:58.2", "31:58.2", "31:58.2", "31:58.3", "31:58.3", "31:58.3", "31:58.4", "31:58.4", "31:58.4", "31:58.5", "31:58.5", "31:58.5", "31:58.6", "31:58.6", "31:58.6", "31:58.7", "31:58.7", "31:58.7", "31:58.8", "31:58.8", "31:58.8", "31:58.9", "31:58.9", "31:58.9", "31:59.0", "31:59.0", "31:59.0", "31:59.1", "31:59.1", "31:59.1", "31:59.2", "31:59.2", "31:59.2", "31:59.3", "31:59.3", "31:59.3", "31:59.4", "31:59.4", "31:59.4", "31:59.5", "31:59.5", "31:59.5", "31:59.6", "31:59.6", "31:59.6", "31:59.7", "31:59.7", "31:59.7", "31:59.8", "31:59.8", "31:59.8", "31:59.9", "31:59.9", "31:59.9", "32:00.0", "32:00.0", "32:00.0", "32:00.1", "32:00.1", "32:00.1", "32:00.2", "32:00.2", "32:00.2", "32:00.3", "32:00.3", "32:00.3", "32:00.4", "32:00.4", "32:00.4", "32:00.5", "32:00.5", "32:00.5", "32:00.6", "32:00.6", "32:00.6", "32:00.7", "32:00.7", "32:00.7", "32:00.8", "32:00.8", "32:00.8", "32:00.9", "32:00.9", "32:00.9", "32:01.0", "32:01.0", "32:01.0", "32:01.1", "32:01.1", "32:01.1", "32:01.2", "32:01.2", "32:01.2", "32:01.3", "32:01.3", "32:01.3", "32:01.4", "32:01.4", "32:01.4", "32:01.5", "32:01.5", "32:01.5", "32:01.6", "32:01.6", "32:01.6", "32:01.7", "32:01.7", "32:01.7", "32:01.8", "32:01.8", "32:01.8", "32:01.9", "32:01.9", "32:01.9", "32:02.0", "32:02.0", "32:02.0", "32:02.1", "32:02.1", "32:02.1", "32:02.2", "32:02.2", "32:02.2", "32:02.3", "32:02.3", "32:02.3", "32:02.4", "32:02.4", "32:02.4", "32:02.5", "32:02.5", "32:02.5", "32:02.6", "32:02.6", "32:02.6", "32:02.7", "32:02.7", "32:02.7", "32:02.8", "32:02.8", "32:02.8", "32:02.9", "32:02.9", "32:02.9", "32:03.0", "32:03.0", "32:03.0", "32:03.1", "32:03.1", "32:03.1", "32:03.2", "32:03.2", "32:03.2", "32:03.3", "32:03.3", "32:03.3", "32:03.4", "32:03.4", "32:03.4", "32:03.5", "32:03.5", "32:03.5", "32:03.6", "32:03.6", "32:03.6", "32:03.7", "32:03.7", "32:03.7", "32:03.8", "32:03.8", "32:03.8", "32:03.9", "32:03.9", "32:03.9", "32:04.0", "32:04.0", "32:04.0", "32:04.1", "32:04.1", "32:04.1", "32:04.2", "32:04.2", "32:04.2", "32:04.3", "32:04.3", "32:04.3", "32:04.4", "32:04.4", "32:04.4", "32:04.5", "32:04.5", "32:04.5", "32:04.6", "32:04.6", "32:04.6", "32:04.7", "32:04.7", "32:04.7", "32:04.8", "32:04.8", "32:04.8", "32:04.9", "32:04.9", "32:04.9", "32:05.0", "32:05.0", "32:05.0", "32:05.1", "32:05.1", "32:05.1", "32:05.2", "32:05.2", "32:05.2", "32:05.3", "32:05.3", "32:05.3", "32:05.4", "32:05.4", "32:05.4", "32:05.5", "32:05.5", "32:05.5", "32:05.6", "32:05.6", "32:05.6", "32:05.7", "32:05.7", "32:05.7", "32:05.8", "32:05.8", "32:05.8", "32:05.9", "32:05.9", "32:05.9", "32:06.0", "32:06.0", "32:06.0", "32:06.1", "32:06.1", "32:06.1", "32:06.2", "32:06.2", "32:06.2", "32:06.3", "32:06.3", "32:06.3", "32:06.4", "32:06.4", "32:06.4", "32:06.5", "32:06.5", "32:06.5", "32:06.6", "32:06.6", "32:06.6", "32:06.7", "32:06.7", "32:06.7", "32:06.8", "32:06.8", "32:06.8", "32:06.9", "32:06.9", "32:06.9", "32:07.0", "32:07.0", "32:07.0", "32:07.1", "32:07.1", "32:07.1", "32:07.2", "32:07.2", "32:07.2", "32:07.3", "32:07.3", "32:07.3", "32:07.4", "32:07.4", "32:07.4", "32:07.5", "32:07.5", "32:07.5", "32:07.6", "32:07.6", "32:07.6", "32:07.7", "32:07.7", "32:07.7", "32:07.8", "32:07.8", "32:07.8", "32:07.9", "32:07.9", "32:07.9", "32:08.0", "32:08.0", "32:08.0", "32:08.1", "32:08.1", "32:08.1", "32:08.2", "32:08.2", "32:08.2", "32:08.3", "32:08.3", "32:08.3", "32:08.4", "32:08.4", "32:08.4", "32:08.5", "32:08.5", "32:08.5", "32:08.6", "32:08.6", "32:08.6", "32:08.7", "32:08.7", "32:08.7", "32:08.8", "32:08.8", "32:08.8", "32:08.9", "32:08.9", "32:08.9", "32:09.0", "32:09.0", "32:09.0", "32:09.1", "32:09.1", "32:09.1", "32:09.2", "32:09.2", "32:09.2", "32:09.3", "32:09.3", "32:09.3", "32:09.4", "32:09.4", "32:09.4", "32:09.5", "32:09.5", "32:09.5", "32:09.6", "32:09.6", "32:09.6", "32:09.7", "32:09.7", "32:09.7", "32:09.8", "32:09.8", "32:09.8", "32:09.9", "32:09.9", "32:09.9", "32:10.0", "32:10.0", "32:10.0", "32:10.1", "32:10.1", "32:10.1", "32:10.2", "32:10.2", "32:10.2", "32:10.3", "32:10.3", "32:10.3", "32:10.4", "32:10.4", "32:10.4", "32:10.5", "32:10.5", "32:10.5", "32:10.6", "32:10.6", "32:10.6", "32:10.7", "32:10.7", "32:10.7", "32:10.8", "32:10.8", "32:10.8", "32:10.9", "32:10.9", "32:10.9", "32:11.0", "32:11.0", "32:11.0", "32:11.1", "32:11.1", "32:11.1", "32:11.2", "32:11.2", "32:11.2", "32:11.3", "32:11.3", "32:11.3", "32:11.4", "32:11.4", "32:11.4", "32:11.5", "32:11.5", "32:11.5", "32:11.6", "32:11.6", "32:11.6", "32:11.7", "32:11.7", "32:11.7", "32:11.8", "32:11.8", "32:11.8", "32:11.9", "32:11.9", "32:11.9", "32:12.0", "32:12.0", "32:12.0", "32:12.1", "32:12.1", "32:12.1", "32:12.2", "32:12.2", "32:12.2", "32:12.3", "32:12.3", "32:12.3", "32:12.4", "32:12.4", "32:12.4", "32:12.5", "32:12.5", "32:12.5", "32:12.6", "32:12.6", "32:12.6", "32:12.7", "32:12.7", "32:12.7", "32:12.8", "32:12.8", "32:12.8", "32:12.9", "32:12.9", "32:12.9", "32:13.0", "32:13.0", "32:13.0", "32:13.1", "32:13.1", "32:13.1", "32:13.2", "32:13.2", "32:13.2", "32:13.3", "32:13.3", "32:13.3", "32:13.4", "32:13.4", "32:13.4", "32:13.5", "32:13.5", "32:13.5", "32:13.6", "32:13.6", "32:13.6", "32:13.7", "32:13.7", "32:13.7", "32:13.8", "32:13.8", "32:13.8", "32:13.9", "32:13.9", "32:13.9", "32:14.0", "32:14.0", "32:14.0", "32:14.1", "32:14.1", "32:14.1", "32:14.2", "32:14.2", "32:14.2", "32:14.3", "32:14.3", "32:14.3", "32:14.4", "32:14.4", "32:14.4", "32:14.5", "32:14.5", "32:14.5", "32:14.6", "32:14.6", "32:14.6", "32:14.7", "32:14.7", "32:14.7", "32:14.8", "32:14.8", "32:14.8", "32:14.9", "32:14.9", "32:14.9", "32:15.0", "32:15.0", "32:15.0", "32:15.1", "32:15.1", "32:15.1", "32:15.2", "32:15.2", "32:15.2", "32:15.3", "32:15.3", "32:15.3", "32:15.4", "32:15.4", "32:15.4", "32:15.5", "32:15.5", "32:15.5", "32:15.6", "32:15.6", "32:15.6", "32:15.7", "32:15.7", "32:15.7", "32:15.8", "32:15.8", "32:15.8", "32:15.9", "32:15.9", "32:15.9", "32:16.0", "32:16.0", "32:16.0", "32:16.1", "32:16.1", "32:16.1", "32:16.2", "32:16.2", "32:16.2", "32:16.3", "32:16.3", "32:16.3", "32:16.4", "32:16.4", "32:16.4", "32:16.5", "32:16.5", "32:16.5", "32:16.6", "32:16.6", "32:16.6", "32:16.7", "32:16.7", "32:16.7", "32:16.8", "32:16.8", "32:16.8", "32:16.9", "32:16.9", "32:16.9", "32:17.0", "32:17.0", "32:17.0", "32:17.1", "32:17.1", "32:17.1", "32:17.2", "32:17.2", "32:17.2", "32:17.3", "32:17.3", "32:17.3", "32:17.4", "32:17.4", "32:17.4", "32:17.5", "32:17.5", "32:17.5", "32:17.6", "32:17.6", "32:17.6", "32:17.7", "32:17.7", "32:17.7", "32:17.8", "32:17.8", "32:17.8", "32:17.9", "32:17.9", "32:17.9", "32:18.0", "32:18.0", "32:18.0", "32:18.1", "32:18.1", "32:18.1", "32:18.2", "32:18.2", "32:18.2", "32:18.3", "32:18.3", "32:18.3", "32:18.4", "32:18.4", "32:18.4", "32:18.5", "32:18.5", "32:18.5", "32:18.6", "32:18.6", "32:18.6", "32:18.7", "32:18.7", "32:18.7", "32:18.8", "32:18.8", "32:18.8", "32:18.9", "32:18.9", "32:18.9", "32:19.0", "32:19.0", "32:19.0", "32:19.1", "32:19.1", "32:19.1", "32:19.2", "32:19.2", "32:19.2", "32:19.3", "32:19.3", "32:19.3", "32:19.4", "32:19.4", "32:19.4", "32:19.5", "32:19.5", "32:19.5", "32:19.6", "32:19.6", "32:19.6", "32:19.7", "32:19.7", "32:19.7", "32:19.8", "32:19.8", "32:19.8", "32:19.9", "32:19.9", "32:19.9", "32:20.0", "32:20.0", "32:20.0", "32:20.1", "32:20.1", "32:20.1", "32:20.2", "32:20.2", "32:20.2", "32:20.3", "32:20.3", "32:20.3", "32:20.4", "32:20.4", "32:20.4", "32:20.5", "32:20.5", "32:20.5", "32:20.6", "32:20.6", "32:20.6", "32:20.7", "32:20.7", "32:20.7", "32:20.8", "32:20.8", "32:20.8", "32:20.9", "32:20.9", "32:20.9", "32:21.0", "32:21.0", "32:21.0", "32:21.1", "32:21.1", "32:21.1", "32:21.2", "32:21.2", "32:21.2", "32:21.3", "32:21.3", "32:21.3", "32:21.4", "32:21.4", "32:21.4", "32:21.5", "32:21.5", "32:21.5", "32:21.6", "32:21.6", "32:21.6", "32:21.7", "32:21.7", "32:21.7", "32:21.8", "32:21.8", "32:21.8", "32:21.9", "32:21.9", "32:21.9", "32:22.0", "32:22.0", "32:22.0", "32:22.1", "32:22.1", "32:22.1", "32:22.2", "32:22.2", "32:22.2", "32:22.3", "32:22.3", "32:22.3", "32:22.4", "32:22.4", "32:22.4", "32:22.5", "32:22.5", "32:22.5", "32:22.6", "32:22.6", "32:22.6", "32:22.7", "32:22.7", "32:22.7", "32:22.8", "32:22.8", "32:22.8", "32:22.9", "32:22.9", "32:22.9", "32:23.0", "32:23.0", "32:23.0", "32:23.1", "32:23.1", "32:23.1", "32:23.2", "32:23.2", "32:23.2", "32:23.3", "32:23.3", "32:23.3", "32:23.4", "32:23.4", "32:23.4", "32:23.5", "32:23.5", "32:23.5", "32:23.6", "32:23.6", "32:23.6", "32:23.7", "32:23.7", "32:23.7", "32:23.8", "32:23.8", "32:23.8", "32:23.9", "32:23.9", "32:23.9", "32:24.0", "32:24.0", "32:24.0", "32:24.1", "32:24.1", "32:24.1", "32:24.2", "32:24.2", "32:24.2", "32:24.3", "32:24.3", "32:24.3", "32:24.4", "32:24.4", "32:24.4", "32:24.5", "32:24.5", "32:24.5", "32:24.6", "32:24.6", "32:24.6", "32:24.7", "32:24.7", "32:24.7", "32:24.8", "32:24.8", "32:24.8", "32:24.9", "32:24.9", "32:24.9", "32:25.0", "32:25.0", "32:25.0", "32:25.1", "32:25.1", "32:25.1", "32:25.2", "32:25.2", "32:25.2", "32:25.3", "32:25.3", "32:25.3", "32:25.4", "32:25.4", "32:25.4", "32:25.5", "32:25.5", "32:25.5", "32:25.6", "32:25.6", "32:25.6", "32:25.7", "32:25.7", "32:25.7", "32:25.8", "32:25.8", "32:25.8", "32:25.9", "32:25.9", "32:25.9", "32:26.0", "32:26.0", "32:26.0", "32:26.1", "32:26.1", "32:26.1", "32:26.2", "32:26.2", "32:26.2", "32:26.3", "32:26.3", "32:26.3", "32:26.4", "32:26.4", "32:26.4", "32:26.5", "32:26.5", "32:26.5", "32:26.6", "32:26.6", "32:26.6", "32:26.7", "32:26.7", "32:26.7", "32:26.8", "32:26.8", "32:26.8", "32:26.9", "32:26.9", "32:26.9", "32:27.0", "32:27.0", "32:27.0", "32:27.1", "32:27.1", "32:27.1", "32:27.2", "32:27.2", "32:27.2", "32:27.3", "32:27.3", "32:27.3", "32:27.4", "32:27.4", "32:27.4", "32:27.5", "32:27.5", "32:27.5", "32:27.6", "32:27.6", "32:27.6", "32:27.7", "32:27.7", "32:27.7", "32:27.8", "32:27.8", "32:27.8", "32:27.9", "32:27.9", "32:27.9", "32:28.0", "32:28.0", "32:28.0", "32:28.1", "32:28.1", "32:28.1", "32:28.2", "32:28.2", "32:28.2", "32:28.3", "32:28.3", "32:28.3", "32:28.4", "32:28.4", "32:28.4", "32:28.5", "32:28.5", "32:28.5", "32:28.6", "32:28.6", "32:28.6", "32:28.7", "32:28.7", "32:28.7", "32:28.8", "32:28.8", "32:28.8", "32:28.9", "32:28.9", "32:28.9", "32:29.0", "32:29.0", "32:29.0", "32:29.1", "32:29.1", "32:29.1", "32:29.2", "32:29.2", "32:29.2", "32:29.3", "32:29.3", "32:29.3", "32:29.4", "32:29.4", "32:29.4", "32:29.5", "32:29.5", "32:29.5", "32:29.6", "32:29.6", "32:29.6", "32:29.7", "32:29.7", "32:29.7", "32:29.8", "32:29.8", "32:29.8", "32:29.9", "32:29.9", "32:29.9", "32:30.0", "32:30.0", "32:30.0", "32:30.1", "32:30.1", "32:30.1", "32:30.2", "32:30.2", "32:30.2", "32:30.3", "32:30.3", "32:30.3", "32:30.4", "32:30.4", "32:30.4", "32:30.5", "32:30.5", "32:30.5", "32:30.6", "32:30.6", "32:30.6", "32:30.7", "32:30.7", "32:30.7", "32:30.8", "32:30.8", "32:30.8", "32:30.9", "32:30.9", "32:30.9", "32:31.0", "32:31.0", "32:31.0", "32:31.1", "32:31.1", "32:31.1", "32:31.2", "32:31.2", "32:31.2", "32:31.3", "32:31.3", "32:31.3", "32:31.4", "32:31.4", "32:31.4", "32:31.5", "32:31.5", "32:31.5", "32:31.6", "32:31.6", "32:31.6", "32:31.7", "32:31.7", "32:31.7", "32:31.8", "32:31.8", "32:31.8", "32:31.9", "32:31.9", "32:31.9", "32:32.0", "32:32.0", "32:32.0", "32:32.1", "32:32.1", "32:32.1", "32:32.2", "32:32.2", "32:32.2", "32:32.3", "32:32.3", "32:32.3", "32:32.4", "32:32.4", "32:32.4", "32:32.5", "32:32.5", "32:32.5", "32:32.6", "32:32.6", "32:32.6", "32:32.7", "32:32.7", "32:32.7", "32:32.8", "32:32.8", "32:32.8", "32:32.9", "32:32.9", "32:32.9", "32:33.0", "32:33.0", "32:33.0", "32:33.1", "32:33.1", "32:33.1", "32:33.2", "32:33.2", "32:33.2", "32:33.3", "32:33.3", "32:33.3", "32:33.4", "32:33.4", "32:33.4", "32:33.5", "32:33.5", "32:33.5", "32:33.6", "32:33.6", "32:33.6", "32:33.7", "32:33.7", "32:33.7", "32:33.8", "32:33.8", "32:33.8", "32:33.9", "32:33.9", "32:33.9", "32:34.0", "32:34.0", "32:34.0", "32:34.1", "32:34.1", "32:34.1", "32:34.2", "32:34.2", "32:34.2", "32:34.3", "32:34.3", "32:34.3", "32:34.4", "32:34.4", "32:34.4", "32:34.5", "32:34.5", "32:34.5", "32:34.6", "32:34.6", "32:34.6", "32:34.7", "32:34.7", "32:34.7", "32:34.8", "32:34.8", "32:34.8", "32:34.9", "32:34.9", "32:34.9", "32:35.0", "32:35.0", "32:35.0", "32:35.1", "32:35.1", "32:35.1", "32:35.2", "32:35.2", "32:35.2", "32:35.3", "32:35.3", "32:35.3", "32:35.4", "32:35.4", "32:35.4", "32:35.5", "32:35.5", "32:35.5", "32:35.6", "32:35.6", "32:35.6", "32:35.7", "32:35.7", "32:35.7", "32:35.8", "32:35.8", "32:35.8", "32:35.9", "32:35.9", "32:35.9", "32:36.0", "32:36.0", "32:36.0", "32:36.1", "32:36.1", "32:36.1", "32:36.2", "32:36.2", "32:36.2", "32:36.3", "32:36.3", "32:36.3", "32:36.4", "32:36.4", "32:36.4", "32:36.5", "32:36.5", "32:36.5", "32:36.6", "32:36.6", "32:36.6", "32:36.7", "32:36.7", "32:36.7", "32:36.8", "32:36.8", "32:36.8", "32:36.9", "32:36.9", "32:36.9", "32:37.0", "32:37.0", "32:37.0", "32:37.1", "32:37.1", "32:37.1", "32:37.2", "32:37.2", "32:37.2", "32:37.3", "32:37.3", "32:37.3", "32:37.4", "32:37.4", "32:37.4", "32:37.5", "32:37.5", "32:37.5", "32:37.6", "32:37.6", "32:37.6", "32:37.7", "32:37.7", "32:37.7", "32:37.8", "32:37.8", "32:37.8", "32:37.9", "32:37.9", "32:37.9", "32:38.0", "32:38.0", "32:38.0", "32:38.1", "32:38.1", "32:38.1", "32:38.2", "32:38.2", "32:38.2", "32:38.3", "32:38.3", "32:38.3", "32:38.4", "32:38.4", "32:38.4", "32:38.5", "32:38.5", "32:38.5", "32:38.6", "32:38.6", "32:38.6", "32:38.7", "32:38.7", "32:38.7", "32:38.8", "32:38.8", "32:38.8", "32:38.9", "32:38.9", "32:38.9", "32:39.0", "32:39.0", "32:39.0", "32:39.1", "32:39.1", "32:39.1", "32:39.2", "32:39.2", "32:39.2", "32:39.3", "32:39.3", "32:39.3", "32:39.4", "32:39.4", "32:39.4", "32:39.5", "32:39.5", "32:39.5", "32:39.6", "32:39.6", "32:39.6", "32:39.7", "32:39.7", "32:39.7", "32:39.8", "32:39.8", "32:39.8", "32:39.9", "32:39.9", "32:39.9", "32:40.0", "32:40.0", "32:40.0", "32:40.1", "32:40.1", "32:40.1", "32:40.2", "32:40.2", "32:40.2", "32:40.3", "32:40.3", "32:40.3", "32:40.4", "32:40.4", "32:40.4", "32:40.5", "32:40.5", "32:40.5", "32:40.6", "32:40.6", "32:40.6", "32:40.7", "32:40.7", "32:40.7", "32:40.8", "32:40.8", "32:40.8", "32:40.9", "32:40.9", "32:40.9", "32:41.0", "32:41.0", "32:41.0", "32:41.1", "32:41.1", "32:41.1", "32:41.2", "32:41.2", "32:41.2", "32:41.3", "32:41.3", "32:41.3", "32:41.4", "32:41.4", "32:41.4", "32:41.5", "32:41.5", "32:41.5", "32:41.6", "32:41.6", "32:41.6", "32:41.7", "32:41.7", "32:41.7", "32:41.8", "32:41.8", "32:41.8", "32:41.9", "32:41.9", "32:41.9", "32:42.0", "32:42.0", "32:42.0", "32:42.1", "32:42.1", 
